vi "Configure External Mixer Enabled.vi"(8 "error in (no error)":errorcluster {"code" format="%.0x"}, 9 "external mixing enabled (Off)":bool, 11 "instrument handle":refnum<k15>) -> (0 "error out":errorcluster {"code" format="%.0x"}, 3 "instrument handle out":refnum<k15>)   [LabVIEW 2009, in "Keysight XSAn.lvlib"]
doc: "This VI enables or disables the external mixer.\n\nSupported Models: All supported"
uses:
  <instrlib>/Keysight XSAn/Keysight XSAn.lvlib
  AgXSAn.dll
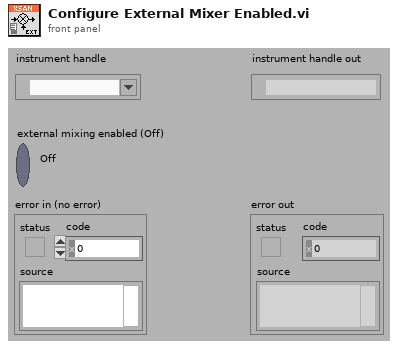
[diagram p1: front panel]
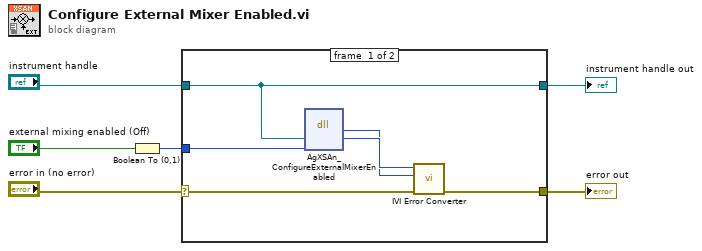
[diagram p0: block diagram]
diagram:
  n1 = Boolean To (0,1)(Boolean="external mixing enabled (Off)") -> (0, 1=w1:i16)
  n2 = case shown="No Error" "error in (no error)" {
    selector: "error in (no error)" -> [w10 w14]
    tunnel: [w11 w14] -> w5
    tunnel: "instrument handle" -> [w8 w13]
    tunnel: [w8 w13] -> w3
    tunnel: w1 -> [w7 _]
    frame #0 {
      n3 = dll-call lib="AgXSAn**.dll" fn="AgXSAn_ConfigureExternalMixerEnabled" ("LabVIEW:IviSpecAn_ConfigureExternalMixerEnabled")("instrument handle"=w8, "external mixing enabled"=w7) -> ("Status"=w9:i32, "instrument handle"=w12:u32)  [unwired: 4 in, 2 out]
      n4 = call <instrlib>:"IVI Error Converter.vi"("error in (no error)"=w10, "IVI error code (0)"=w9, "instrument handle"=w12) -> ("error out"=w11:errorcluster)  [unwired: 7 in, 1 out]
    }
    frame #1 {
    }
  }
  "error out" <- w5
  "instrument handle out" <- w3
